vi "02 - Simple Connection to Serial COM.vi"() -> ()   [LabVIEW 2026]
uses:
  <vilib>/Instr/_visa.llb/VISA Configure Serial Port (Instr).vi
  <extravilib>/ChannelInstances/Tag-bool/Instantiate.vi
  <extravilib>/ChannelInstances/Tag-bool/EndpointRead.vi
  <extravilib>/ChannelInstances/Tag-bool/Endpoint.vi
  <extravilib>/ChannelInstances/Tag-bool.lvlib
panel:
  out "Numeric 2":i32
  out "Numeric":i32
  out "Response":string
  in  "VISA resource name 2":refnum<visa-resource-name>="COM20"
  in  "Termination Character":u8=10 format="%.0x"
  in  "End Write on Termination Character?":bool=TRUE
  in  "VISA resource name":refnum<visa-resource-name>="COM19"
  in  "End Read on Termination Character?":bool=TRUE
  in  "Command":string="*IDN?"
  in  "Stop":bool
  in  "Write":bool
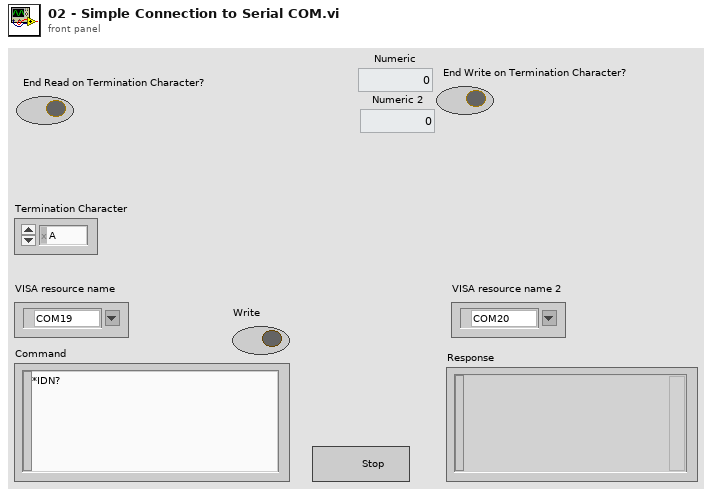
[diagram p1: front panel]
types:
  T1 = typedef "Tag-bool.lvlib/))Channel.ctl" = refnum<queue>
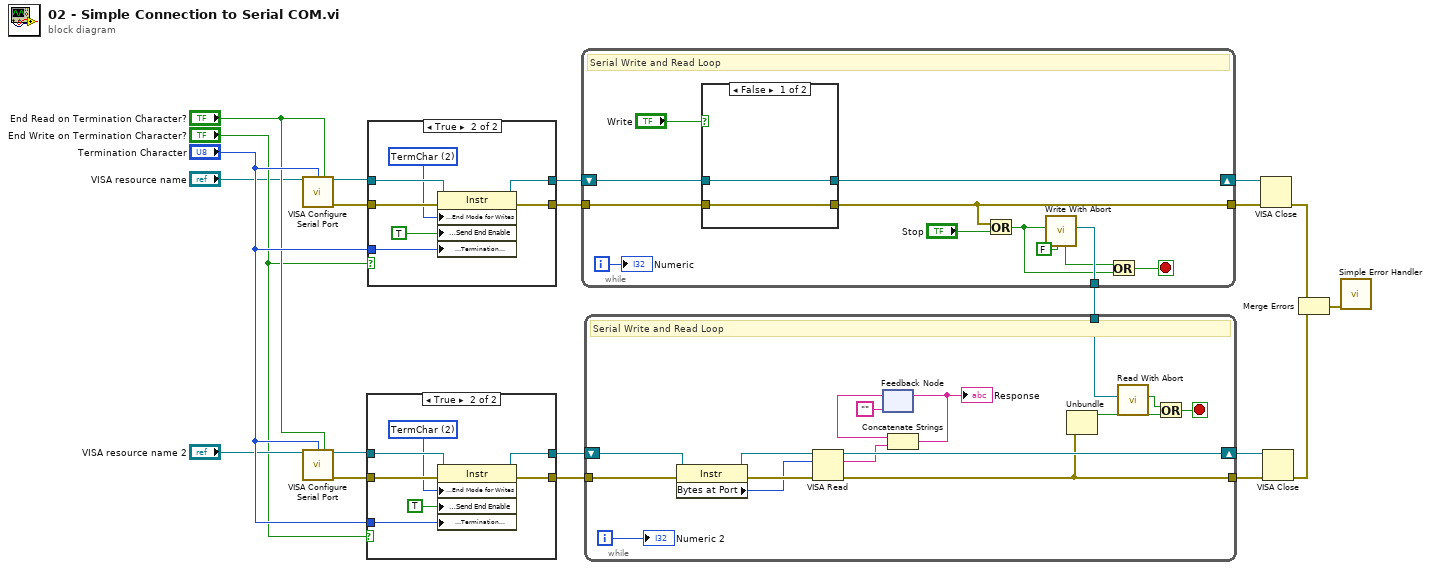
[diagram p0: block diagram]
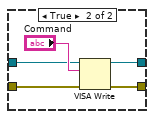
[diagram p3: hidden frame]
diagram:
  n1 = call-poly "VISA Configure Serial Port"("VISA resource name"="VISA resource name", "termination char\n(0xA = '\\n' = LF)"="Termination Character", "Enable Termination\nChar (T)"="End Read on Termination Character?") -> ("VISA resource name out"=w13:refnum<visa-resource-name>, "error out"=w20:errorcluster)  [unwired: 7 in, 4 out]
  n2 = call-poly "VISA Configure Serial Port"("VISA resource name"="VISA resource name 2", "termination char\n(0xA = '\\n' = LF)"="Termination Character", "Enable Termination\nChar (T)"="End Read on Termination Character?") -> ("VISA resource name out"=w10:refnum<visa-resource-name>, "error out"=w17:errorcluster)  [unwired: 7 in, 4 out]
  n3 = case shown="True" "End Write on Termination Character?" {
    tunnel: w10 -> [w22 w25]
    tunnel: w17 -> [w23 w30]
    tunnel: [w22 w26] -> w11
    tunnel: [w23 w29] -> w18
    tunnel: "Termination Character" -> [_ w28]
    frame False {
    }
    frame True {
      w24 = u16 2 items=["None", "LastBit", "TermChar", "Break"] ("Serial Settings:Serial End Mode for Writes")
      n4 = property class="Instr"(reference=w25, error in=w30, "Serial Settings:End Mode for Writes"=w24, "Message Based Settings:Send End Enable"=TRUE, "Message Based Settings:Termination Character"=w28) -> (reference out=w26:refnum<visa-resource-name>, error out=w29:errorcluster)
    }
  }
  n5 = case shown="True" "End Write on Termination Character?" {
    tunnel: w13 -> [w31 w36]
    tunnel: w20 -> [w32 w39]
    tunnel: [w31 w35] -> w12
    tunnel: [w32 w38] -> w19
    tunnel: "Termination Character" -> [_ w37]
    frame False {
    }
    frame True {
      w33 = u16 2 items=["None", "LastBit", "TermChar", "Break"] ("Serial Settings:Serial End Mode for Writes")
      n6 = property class="Instr"(reference=w36, error in=w39, "Serial Settings:End Mode for Writes"=w33, "Message Based Settings:Send End Enable"=TRUE, "Message Based Settings:Termination Character"=w37) -> (reference out=w35:refnum<visa-resource-name>, error out=w38:errorcluster)
    }
  }
  n7 = while {
    shift-right: [w48] -> w14
    shift-left: w12 -> [w49]
    tunnel: w19 -> [w51]
    tunnel: [w50] -> w21
    tunnel: [w45] -> w5
    i -> [w40]
    stop <- w41 stop-if-true
    # "Serial Write and Read Loop"
    n8 = case shown="False" "Write" {
      tunnel: w49 -> [w52 w55]
      tunnel: w51 -> [w53 w58]
      tunnel: [w52 w54] -> w48
      tunnel: [w53 w57] -> w50
      frame False {
      }
      frame True {
        n9 = VISA Write(VISA resource name=w55, write buffer="Command", error in (no error)=w58) -> (VISA resource name out=w54:refnum<visa-resource-name>, error out=w57:errorcluster)  [unwired: 1 out]
      }
    }
    n10 = Or(x=w50, y="Stop") -> (x .or. y?=w43:bool)
    n11 = call <extravilib>:"Write With Abort.vi"("abort"=FALSE, "element"=w43) -> ("channel"=w45:T1, "aborted?"=w42:bool)  [unwired: 7 in, 1 out]
    n12 = Or(x=w42, y=w43) -> (x .or. y?=w41:bool)
    "Numeric" <- w40
  }
  n13 = while {
    shift-right: [w74] -> w9
    shift-left: w11 -> [w62]
    tunnel: w18 -> [w75]
    tunnel: [w72] -> w16
    tunnel: w5 -> [w73]
    i -> [w59]
    stop <- w68 stop-if-true
    # "Serial Write and Read Loop"
    n14 = property class="Instr"(reference=w62, error in=w75) -> (reference out=w61:refnum<visa-resource-name>, error out=w63:errorcluster, "Bytes at Port"=w60:u32)
    n15 = VISA Read(VISA resource name=w61, byte count=w60, error in (no error)=w63) -> (VISA resource name out=w74:refnum<visa-resource-name>, read buffer=w67:string, error out=w72:errorcluster)  [unwired: 1 out]
    n16 = feedback #1("") -> (w66:string)
    n17 = Concatenate Strings(w66, w67) -> (w65:string)
    "Response" <- w65
    n18 = feedback-in #1(w65) -> ()
    n19 = Unbundle(w72) -> ("status"=w71:bool)  [unwired: 2 out]
    n20 = call <extravilib>:"Read With Abort.vi"("abort"=w71, "channel"=w73) -> ("element"=w70:bool, "aborted?"=w69:bool)  [unwired: 7 in, 1 out]
    n21 = Or(x=w70, y=w69) -> (x .or. y?=w68:bool)
    "Numeric 2" <- w59
  }
  n22 = VISA Close(VISA resource name=w14, error in (no error)=w21) -> (error out=w4:errorcluster)
  n23 = VISA Close(VISA resource name=w9, error in (no error)=w16) -> (error out=w3:errorcluster)
  n24 = Merge Errors(w4, w3) -> (w2:errorcluster)
  n25 = call <vilib>:"Simple Error Handler.vi"("error in (no error)"=w2) -> ()  [unwired: 1 in, 8 out]
